vi "PCP SIC Command Q.vi"(11 "error in (no error)":errorcluster) -> (8 "PCP cmd Q":refnum<queue>, 15 "error out":errorcluster)   [LabVIEW 2011]
uses:
  PCP Command definer.ctl
  PCP Commands.ctl
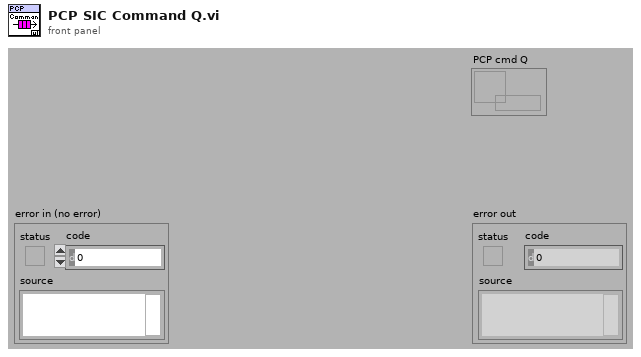
[diagram p1: front panel]
types:
  T1 = typedef "PCP Command definer.ctl" = cluster{"Action":T2, "n(0)":i32, "d(0.0)":dbl}
  T2 = typedef "PCP Commands.ctl" = enum16{"do not use HE - Help", "RDd - Most used inputs", "RA - All analog inputs", "RE n Reset DO n", "SE n Set DO n", "RP - Get digital inputs", "VA d Set AO A  Motor Volt", "VB d Set AO B  Cable Resistance", "VEr - Get Version", "DYp - Depth counter", "DR - Reset Depth Counter", "DS n Set Depth options(0-3)", "do not use ME - Manual mode enabled", "MD - Manual mode disabled", "ID - Get ID(2001)", "TS - Get Timestamp", "TO d(s)  Set timeout", "do not use LO n Start Loop Mode(1,2)", "AL n RD&LO variation", "ST - Stop Loop Mode"}
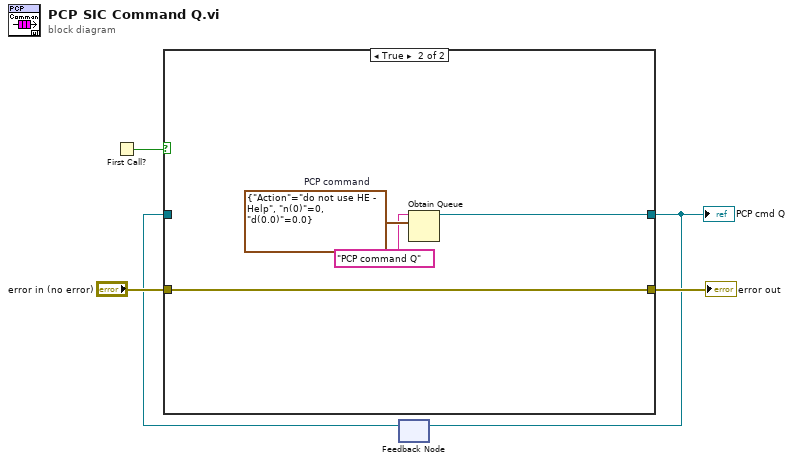
[diagram p0: block diagram]
diagram:
  n1 = First Call?() -> (First Call?: T/F=w3:bool)
  n2 = feedback #1() -> (w1:refnum<queue>)  [unwired: 1 in]
  n3 = case shown="True" w3 {
    tunnel: [w7 w11] -> w5
    tunnel: "error in (no error)" -> [w7 w11]
    tunnel: [w6 w8] -> w2
    tunnel: w1 -> [w6 _]
    frame False {
    }
    frame True {
      w10 = T1 {"Action"=enum."do not use HE - Help", "n(0)"=0, "d(0.0)"=0.0}  # PCP command
      n4 = Obtain Queue(name (unnamed)="PCP command Q", element data type=w10) -> (queue out=w8:refnum<queue>)  [unwired: 3 in, 2 out]
    }
  }
  "error out" <- w5
  "PCP cmd Q" <- w2
  n5 = feedback-in #1(w2) -> ()
